vi "MsgFF.vi"(8 "error in":errorcluster, 11 "Data":u8[](array[numeric]) format="%02x") -> (0 "error out":errorcluster, 2 "CF_Count":i32, 3 "FF_DL":i32)   [LabVIEW 2011, in "Konvolucio MUDS150628.lvlib"]
uses:
  <instrlib>/Konvolucio MUDS150628/Konvolucio MUDS150628.lvlib
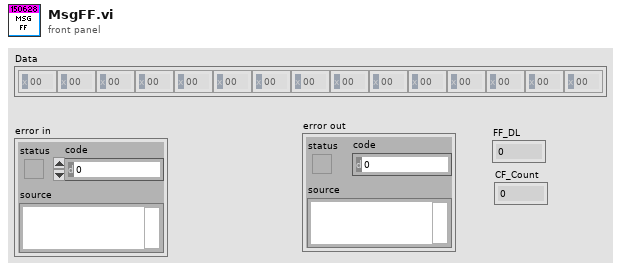
[diagram p1: front panel]
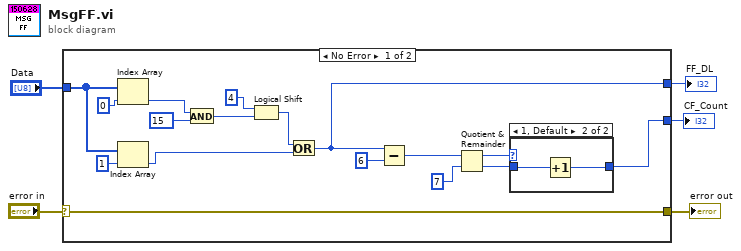
[diagram p0: block diagram]
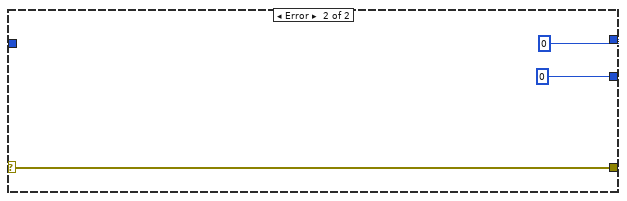
[diagram p3: hidden frame]
diagram:
  n1 = case shown="No Error" "error in" {
    selector: "error in" -> [w7 w28]
    tunnel: [w21 0] -> w5
    tunnel: [w16 0] -> w4
    tunnel: [w7 w28] -> w2
    tunnel: "Data" -> [w6 _]
    frame No Error {
      n2 = Index Array(array=w6, index=0) -> (element=w11:u8)
      n3 = Index Array(array=w6, index=1) -> (element=w14:u8)
      n4 = And(x=w11, y=15) -> (x .and. y?=w13:i32)
      n5 = Logical Shift(y=i8 4, x=w13) -> (x << y=w15:i32)
      n6 = Or(x=w15, y=w14) -> (x .or. y?=w16:i32)
      n7 = Subtract(x=w16, y=6) -> (x-y=w22:i32)
      n8 = Quotient & Remainder(x=w22, y=7) -> (x-y*floor(x/y)=w19:i32, floor(x/y)=w20:i32)
      n9 = case shown="1, Default" w19 {
        tunnel: [w23 w24] -> w21
        tunnel: w20 -> [w23 w25]
        frame 0 {
        }
        frame 1, Default {
          n10 = Increment(x=w25) -> (x+1=w24:i32)
        }
      }
    }
    frame Error {
    }
  }
  "FF_DL" <- w4
  "CF_Count" <- w5
  "error out" <- w2
